vi "Configure Noise.vi"(0 "VISA resource name":refnum<visa-resource-name>, 1 "Enable BandSet (T:Enable)":bool=TRUE, 5 "Channel (1:Channel 1)":i32(ring)=1 items=["Channel 1"=1, "Channel 2"=2], 7 "BandWidth (80 MHz)":dbl=80000000.0 format="%#.3g", 9 "Mean (0.00 V)":dbl min=-9.996 max=9.996 format="%#.3g", 11 "error in (no error)":errorcluster, 12 "Standard Deviation (0.008 V)":dbl=0.008 format="%#.4g") -> (4 "VISA resource name out":refnum<visa-resource-name>, 15 "error out":errorcluster)   [LabVIEW 2023, in "Siglent SDG X Series.lvlib"]
doc: "Configures Noise waveform and parameters."
uses:
  Siglent SDG X Series.lvlib
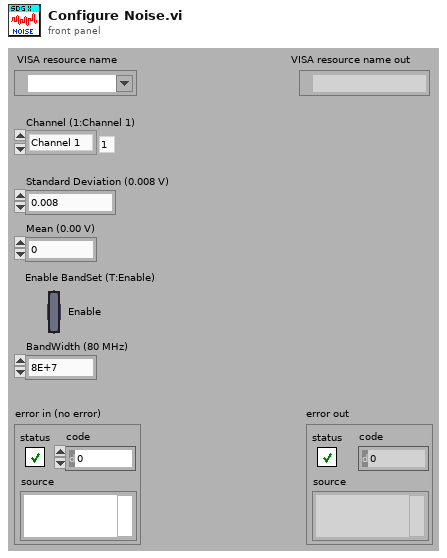
[diagram p1: front panel]
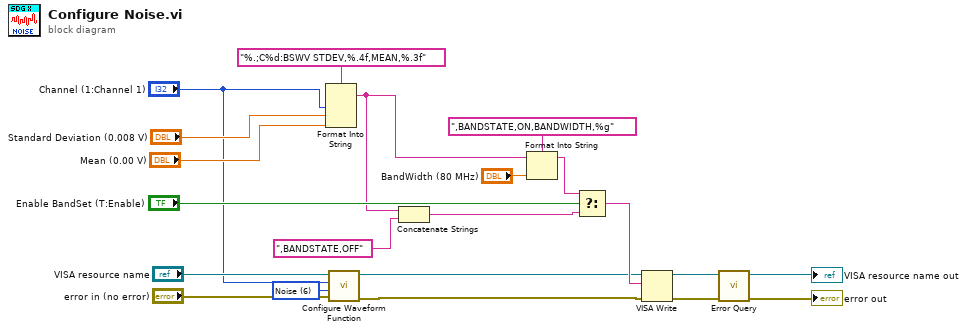
[diagram p0: block diagram]
diagram:
  w1 = u16 6 items=["Sine", "Square", "Ramp", "DC", "Pulse", "Arb", "Noise", "PRBS", "IQ"] ("Waveform Function (0: Sine)")
  n1 = Format Into String(format string="%.;C%d:BSWV STDEV,%.4f,MEAN,%.3f", "Channel (1:Channel 1)", "Standard Deviation (0.008 V)", "Mean (0.00 V)") -> (resulting string=w8:string)  [unwired: 2 in, 1 out]
  n2 = call "Configure Waveform Function.vi"("error in (no error)"="error in (no error)", "Waveform Function (0: Sine)"=w1, "Channel (1:Channel 1)"="Channel (1:Channel 1)", "VISA resource name"="VISA resource name") -> ("error out"=w3:errorcluster, "VISA resource name out"=w4:refnum<visa-resource-name>)  [unwired: 6 in]
  n3 = Concatenate Strings(w8, ",BANDSTATE,OFF" ("格式字符串")) -> (w7:string)
  n4 = Format Into String(format string=",BANDSTATE,ON,BANDWIDTH,%g" ("格式字符串"), initial string=w8, "BandWidth (80 MHz)") -> (resulting string=w11:string)  [unwired: 1 in, 1 out]
  n5 = Select(t=w11, s="Enable BandSet (T:Enable)", f=w7) -> (s? t:f=w10:string)
  n6 = VISA Write(VISA resource name=w4, write buffer=w10, error in (no error)=w3) -> (VISA resource name out=w21:refnum<visa-resource-name>, error out=w20:errorcluster)  [unwired: 1 out]
  n7 = call "Error Query.vi"("error in (no error)"=w20, "VISA resource name"=w21) -> ("error out"=→"error out":errorcluster, "VISA resource name out"=→"VISA resource name out":refnum<visa-resource-name>)  [unwired: 6 in, 2 out]
